vi "main - incasm.vi"() -> ()   [LabVIEW 2025]
uses:
  incASM/incrASM.dll
panel:
  out "pass":bool
  out "ASM DLL":dbl
  out "LabVIEW":dbl
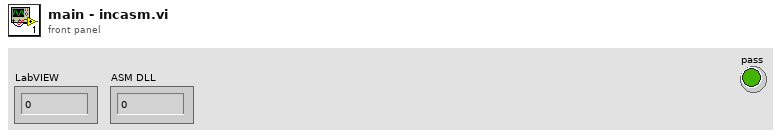
[diagram p1: front panel]
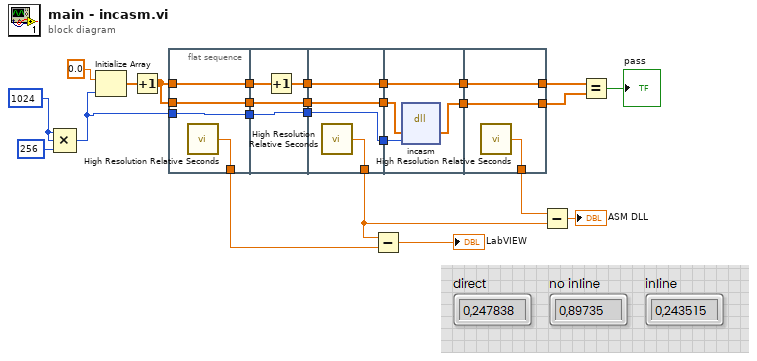
[diagram p0: block diagram]
diagram:
  w24 = 1024
  n1 = Compound Arithmetic op=MULTIPLY(w24, w24, 256 ("value")) -> (w4:i32)
  n2 = Initialize Array(0.0 ("element"), w4) -> (w14:dbl[])
  n3 = Increment(x=w14) -> (x+1=w9:dbl[])
  n4 = flat-sequence {
    tunnel: [w29] -> w23
    tunnel: w9 -> [w29]
    tunnel: [w28] -> w17
    tunnel: [w27] -> w10
    tunnel: w9 -> [w27]
    tunnel: [w26] -> w5
    tunnel: w4 -> [w26]
    tunnel: w23 -> [w33]
    tunnel: [w32] -> w22
    tunnel: [w31] -> w11
    tunnel: w10 -> [w31]
    tunnel: [w30] -> w6
    tunnel: w5 -> [w30]
    tunnel: w22 -> [w37]
    tunnel: [w37] -> w21
    tunnel: [w36] -> w18
    tunnel: [w35] -> w12
    tunnel: w11 -> [w35]
    tunnel: [w34] -> w7
    tunnel: w6 -> [w34]
    tunnel: w21 -> [w41]
    tunnel: [w41] -> w20
    tunnel: w12 -> [w40]
    tunnel: w7 -> [w39]
    tunnel: [w38] -> w3
    tunnel: w20 -> [w43]
    tunnel: [w44] -> w19
    tunnel: [w43] -> w8
    tunnel: [w42] -> w2
    tunnel: w3 -> [w42]
    frame #0 {
      n5 = call <vilib>:"High Resolution Relative Seconds.vi"() -> ("relative seconds"=w28:dbl)
    }
    frame #1 {
      n6 = Increment(x=w33) -> (x+1=w32:dbl[])
    }
    frame #2 {
      n7 = call <vilib>:"High Resolution Relative Seconds.vi"() -> ("relative seconds"=w36:dbl)
    }
    frame #3 {
      n8 = dll-call lib="C:/Users/108003658/OneDrive - Baker Hughes/Desktop/incASM/incrASM.dll" fn="incasm"("arg1"=w40, "size"=w39) -> ("arg1"=w38:dbl[])  [unwired: 5 in, 2 out]
    }
    frame #4 {
      n9 = call <vilib>:"High Resolution Relative Seconds.vi"() -> ("relative seconds"=w44:dbl)
    }
  }
  n10 = Subtract(x=w18, y=w17) -> (x-y=→"LabVIEW":dbl)
  n11 = Subtract(x=w19, y=w18) -> (x-y=→"ASM DLL":dbl)
  n12 = Equal?(x=w8, y=w2) -> (x = y?=→"pass":bool)
